vi "Lev-Mar abx.vi"(0 "X":dbl[](array[numeric]) format="%0.2f", 1 "Y":dbl[](array[numeric]) format="%0.2f", 2 "Coefficients":dbl[](array[numeric]) format="%0.2f", 3 "Standard Deviation":dbl[](array[numeric]) format="%0.2f", 4 "derivative":T1(ring)) -> (5 "Alpha":dbl[][](array[numeric]) format="%0.2f", 6 "Beta":dbl[](array[numeric]) format="%0.2f", 7 "chiSqr":dbl format="%0.2f")   [LabVIEW 2018, in "NI_AALPro.lvlib"]
uses:
  NI_AALPro.lvlib
panel:
  # "Lev-Mar\nabx"
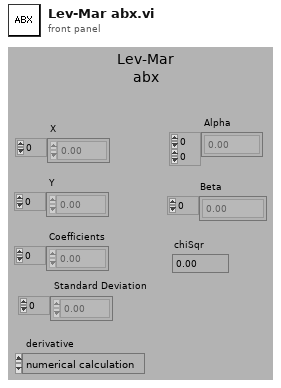
[diagram p1: front panel]
types:
  T1 = enum32{"numerical calculation", "formula calculation"}
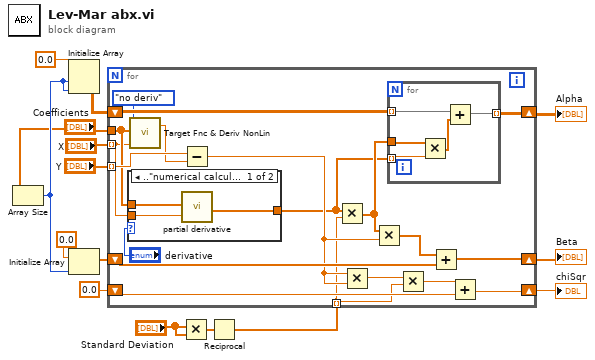
[diagram p0: block diagram]
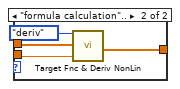
[diagram p2: hidden frame]
diagram:
  n1 = Array Size(array="Coefficients") -> (size(s)=w13:i32)
  n2 = Initialize Array(0.0, w13, w13) -> (w11:dbl[][])
  n3 = Initialize Array(0.0, w13) -> (w12:dbl[])
  n4 = Multiply(x="Standard Deviation", y="Standard Deviation") -> (x*y=w3:dbl[])
  n5 = Reciprocal(x=w3) -> (1/x=w1:dbl[])
  n6 = for {
    tunnel: "X" -> [w22] mode=indexing
    shift-right: [w29] -> w9
    shift-left: w12 -> [w31]
    shift-right: [w26] -> w6
    shift-left: w11 -> [w27]
    shift-right: [w25] -> w2
    shift-left: 0.0 -> [w33]
    tunnel: "Y" -> [w32] mode=indexing
    tunnel: "Coefficients" -> [w23]
    tunnel: w1 -> [w17] mode=indexing
    n7 = case shown="..\"numerical calculation\"" "derivative" {
      tunnel: [w35 w41] -> w16
      tunnel: w23 -> [w37 w40]
      tunnel: w22 -> [w36 w39]
      frame .."numerical calculation" {
        n8 = call "partial derivative.vi"("x"=w36, "Coefficients"=w37) -> ("Partial Derivative"=w35:dbl[])
      }
      frame "formula calculation".. {
        n9 = call "Target Fnc & Deriv NonLin.vi"("X"=w39, "Coefficients"=w40, "Flag"=enum16{"no deriv", "deriv"}."deriv") -> ("Derivatives"=w41:dbl[])  [unwired: 1 out]
      }
    }
    n10 = call "Target Fnc & Deriv NonLin.vi"("X"=w22, "Coefficients"=w23, "Flag"=enum16{"no deriv", "deriv"}."no deriv") -> ("Y"=w24:dbl)  [unwired: 1 out]
    n11 = Subtract(x=w32, y=w24) -> (x-y=w28:dbl)
    n12 = Multiply(x=w16, y=w17) -> (x*y=w19:dbl[])
    n13 = Multiply(x=w28, y=w28) -> (x*y=w34:dbl)
    n14 = Multiply(x=w19, y=w28) -> (x*y=w30:dbl[])
    n15 = for {
      tunnel: w19 -> [w46]
      tunnel: w27 -> [w45] mode=indexing
      tunnel: [w43] -> w26 mode=indexing
      tunnel: w16 -> [w42] mode=indexing
      n16 = Multiply(x=w46, y=w42) -> (x*y=w44:dbl[])
      n17 = Add(x=w45, y=w44) -> (x+y=w43:dbl[])
    }
    n18 = Multiply(x=w34, y=w17) -> (x*y=w18:dbl)
    n19 = Add(x=w30, y=w31) -> (x+y=w29:dbl[])
    n20 = Add(x=w18, y=w33) -> (x+y=w25:dbl)
  }
  "Alpha" <- w6
  "Beta" <- w9
  "chiSqr" <- w2
